vi "Radians to Pulses.vi"(1 "gear ratio":dbl, 2 "angle (rad)":dbl) -> (0 "encoder pulses":i32)   [LabVIEW 2011]
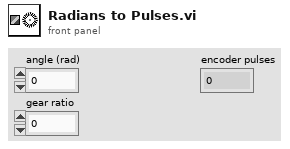
[diagram p1: front panel]
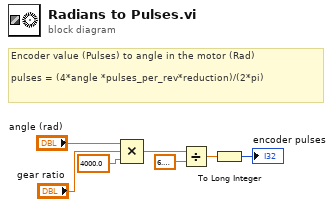
[diagram p0: block diagram]
diagram:
  # "Encoder value (Pulses) to angle in the motor (Rad)\n\npulses = (4*angle *pulses_per_rev*reduction)/(2*pi)"
  n1 = Compound Arithmetic op=MULTIPLY("angle (rad)", "gear ratio", 4000.0 ("x")) -> (w3:dbl)
  n2 = Divide(x=w3, y=6.283185307179586) -> (x/y=w1:dbl)
  n3 = To Long Integer(number=w1) -> (32bit integer=→"encoder pulses":i32)
